vi "Clean Builds.vi"() -> ()   [LabVIEW 2010]
panel:
  out "error out":errorcluster
  in  "Build folder prefix":string="Build #"
  out "Progress":u8(slide) scale=0.0..100.0
  out "Builds deleted":u32
  in  "# to keep":i32=5
  in  "Builds":path=path "C:/Builds"
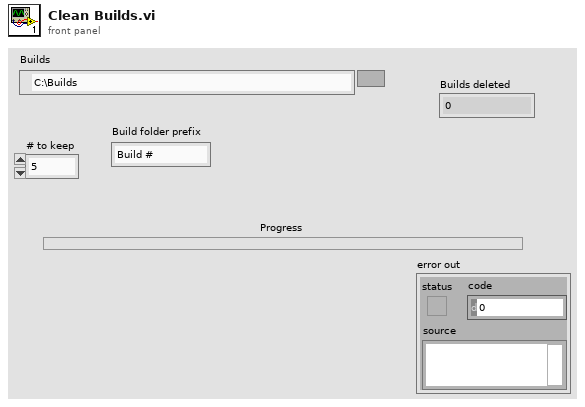
[diagram p1: front panel]
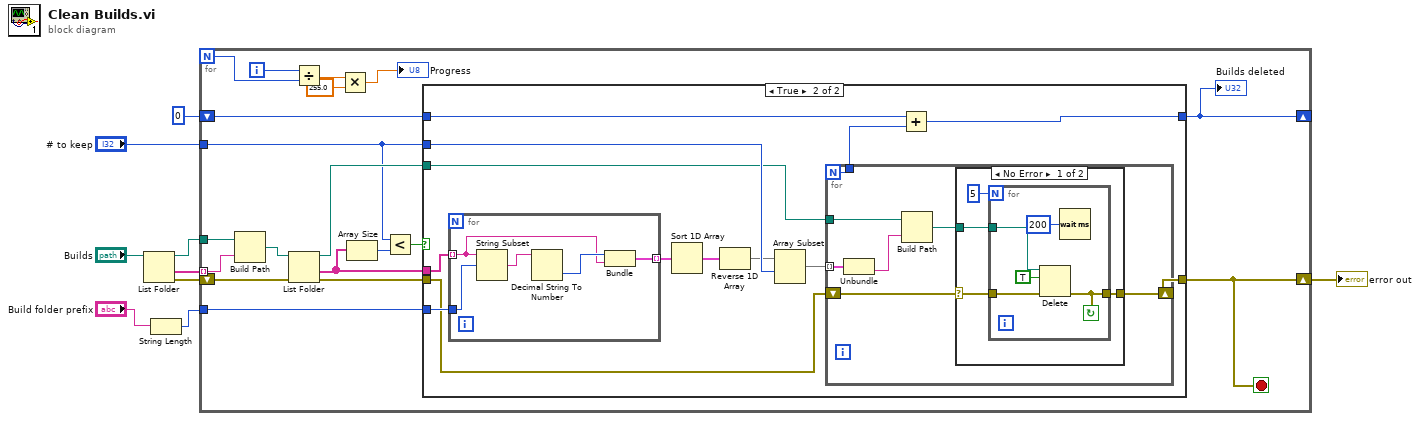
[diagram p0: block diagram]
diagram:
  n1 = List Folder(path="Builds") -> (path out=w7:path, folder names=w8:string[], error out=w9:errorcluster)  [unwired: 3 in, 1 out]
  n2 = String Length(string="Build folder prefix") -> (length=w4:i32)
  n3 = for {
    N -> [w17]
    shift-right: [w10] -> w2
    shift-left: w9 -> [w26]
    tunnel: w8 -> [w28] mode=indexing
    tunnel: w7 -> [w27]
    tunnel: "# to keep" -> [w18]
    tunnel: w4 -> [w19]
    shift-right: [w11] -> _
    shift-left: u32 0 ("y") -> [w12]
    i -> [w16]
    stop <- w10 stop-if-true
    n4 = Build Path(base path=w27, name or relative path=w28) -> (appended path=w25:path)
    n5 = List Folder(path=w25, error in=w26) -> (path out=w20:path, folder names=w21:string[], error out=w22:errorcluster)  [unwired: 2 in, 1 out]
    n6 = Divide(x=w16, y=w17) -> (x/y=w15:dbl)
    n7 = Multiply(x=w15, y=255.0) -> (x*y=→"Progress":dbl)
    n8 = Array Size(array=w21) -> (size(s)=w24:i32)
    n9 = Less?(x=w18, y=w24) -> (x < y?=w23:bool)
    n10 = case shown="True" w23 {
      tunnel: w22 -> [w30 w36]
      tunnel: w21 -> [_ w43]
      tunnel: w20 -> [_ w37]
      tunnel: w19 -> [_ w42]
      tunnel: w18 -> [_ w39]
      tunnel: [w30 w35] -> w10
      tunnel: w12 -> [w29 w33]
      tunnel: [w29 w32] -> w11
      frame False {
      }
      frame True {
        n11 = for {
          tunnel: w43 -> [w62] mode=indexing
          tunnel: w42 -> [w65]
          tunnel: [w61] -> w41 mode=indexing
          n12 = String Subset(string=w62, offset (0)=w65) -> (substring=w64:string)  [unwired: 1 in]
          n13 = Decimal String To Number(string=w64) -> (number=w63:i32)  [unwired: 2 in, 1 out]
          n14 = Bundle(w63, w62) -> (w61:cluster{i32, string})  [unwired: 1 in]
        }
        n15 = Sort 1D Array(array=w41) -> (sorted array=w40:cluster{i32, string}[])
        n16 = Reverse 1D Array(array=w40) -> (reversed array=w31:cluster{i32, string}[])
        n17 = Array Subset(array=w31, index=w39) -> (w38:cluster{i32, string}[])  [unwired: 1 in]
        n18 = for {
          N -> [w45]
          tunnel: w38 -> [w50] mode=indexing
          tunnel: w37 -> [w49]
          shift-right: [w46] -> w35
          shift-left: w36 -> [w44]
          tunnel: [w45] -> w34
          n19 = Unbundle(w50) -> (w48:string)  [unwired: 1 out]
          n20 = Build Path(base path=w49, name or relative path=w48) -> (appended path=w47:path)
          n21 = case shown="No Error" w44 {
            selector: w44 -> [w51 w60]
            tunnel: w47 -> [w54 _]
            tunnel: [w53 w60] -> w46
            frame No Error {
              n22 = for {
                N: 5 -> [_]
                tunnel: w51 -> [w59]
                tunnel: w54 -> [w58]
                tunnel: [w56] -> w53
                stop <- w56 continue-if-true
                n23 = Delete(path (use dialog)=w58, entire hierarchy (F)=TRUE, error in=w59) -> (error out=w56:errorcluster)  [unwired: 2 in, 2 out]
                n24 = Wait (ms)(milliseconds to wait=u32 200) -> ()  [unwired: 1 out]
              }
            }
            frame Error {
            }
          }
        }
        n25 = Add(x=w33, y=w34) -> (x+y=w32:u32)
      }
    }
    "Builds deleted" <- w11
  }
  "error out" <- w2
